vi "Create Structure ID from Structure.vi"(9 "Alphabet":string[](array[string])=["0", "1", "2", "3", "4", "5", "6", "7", "8", "9", "a", "b", "c", "d", "e", "f", "g", "h", "i", "j", "k", "l", "m", "n", "o", "p", "q", "r", "s", "t", "u", "v", "w", "x", "y", "z", "A", "B", "C", "D", "E", "F", "G", "H", "I", "J", "K", "L", "M", "N", "O", "P", "Q", "R", "S", "T", "U", "V", "W", "X", "Y", "Z"], 10 "ID Length":i32=12, 11 "Structure":T1={"Structure ID"="A3B3_strain", "Lattice vector a"=[4.67354, 0.0, 0.0], "Lattice vector b"=[0.0, 8.0948, 0.0], "Lattice vector c"=[0.0, 0.0, 23.043272], "Atoms Array"=[{"Atom Name"="Cd", "Positions (Direct)"=[[0.0, 0.3333526109234154, 0.0418710942225006], [0.5000009999999975, 0.8333529332228705, 0.0418710547186735], [0.5000009999999975, 0.166659409006074, 0.20845808075038], [0.0, 0.6666596363811387, 0.2084580241418204], [0.0, -8.44898704729e-05, 0.3751631556991639], [0.5000009999999975, 0.4999164138500652, 0.375163134357792], [0.0, 8.44898704729e-05, 0.8751631556991638], [0.5000009999999975, 0.5000855861499368, 0.8751631343577921], [0.0, 0.3333423636188632, 0.7084570241418229], [0.5000009999999975, 0.833342590993928, 0.7084570807503824], [0.5000009999999975, 0.1666490667771315, 0.5418710547186734], [0.0, 0.6666493890765864, 0.5418710942225006]], "Positions (Cartesian)"=[[0.0, 2.6984227149028626, 0.9648470131067098], [2.3367746735399884, 6.7458253238524915, 0.9648461028092771], [2.3367746735399884, 1.3490745840223677, 4.803556255328971], [0.0, 5.396476424578041, 4.803554950882535], [0.0, -0.0006839286035040309, 8.644986641154185], [2.3367746735399884, 4.0467233868335075, 8.644986149379148], [0.0, 0.0006839286035040309, 20.166622641154184], [2.3367746735399884, 4.048092802766508, 20.16662214937915], [0.0, 2.6983397650219736, 16.32516790761059], [2.3367746735399884, 6.745741605577648, 16.325169212057027], [2.3367746735399884, 1.348990865747524, 12.486482102809275], [0.0, 5.396393474697152, 12.48648301310671]]}, {"Atom Name"="Te", "Positions (Direct)"=[[0.0, 0.9999785268032801, -4.68232631346e-05], [0.5000009999999975, 0.4999797936920724, -4.67924585214e-05], [0.0, 0.3333755265141826, 0.1664730611888124], [0.5000009999999975, 0.8333756986686149, 0.1664729662126494], [0.5000009999999975, 0.1665154827798591, 0.3330835443926201], [0.0, 0.6665158170693574, 0.3330835000372194], [0.0, 0.3334861829306446, 0.833082500037222], [0.5000009999999975, 0.833486517220143, 0.8330825443926226], [0.5000009999999975, 0.16662630133138, 0.6664729662126494], [0.0, 0.6666264734858195, 0.6664730611888123], [0.0, 2.14731967198e-05, 0.4999531767368653], [0.5000009999999975, 0.5000222063079295, 0.4999532075414786]], "Positions (Cartesian)"=[[0.0, 8.094626178767191, -0.0010789611883381606], [2.3367746735399884, 4.047236433978587, -0.0010782513492573382], [0.0, 2.6986082120270054, 3.8360840296464476], [2.3367746735399884, 6.746009605582704, 3.8360818410848903], [2.3367746735399884, 1.3479095300064032, 7.67533471216322], [0.0, 5.395312236013034, 7.675333690069658], [0.0, 2.6995039535869814, 19.196946646797716], [2.3367746735399884, 6.746906659593613, 19.19694766889128], [2.3367746735399884, 1.3488065840172547, 15.357717841084892], [0.0, 5.396207977573011, 15.357720029646448], [0.0, 0.00017382123280743704, 11.52055703881166], [2.3367746735399884, 4.0475797556214275, 11.520557748650743]]}], "# of atoms"=24}) -> (3 "Structure ID":string="S9HVHL68rkOYQr")   [LabVIEW 2010]
uses:
  <vilib>/Analysis/_algsub.llb/Real Vector Norm.vi
  <vilib>/Analysis/NI_AALPro.lvlib
panel:
  out "Numeric 2":dbl=27.85452959635157
  out "Numeric":dbl=0.1091853688299409 format="%#_12g"
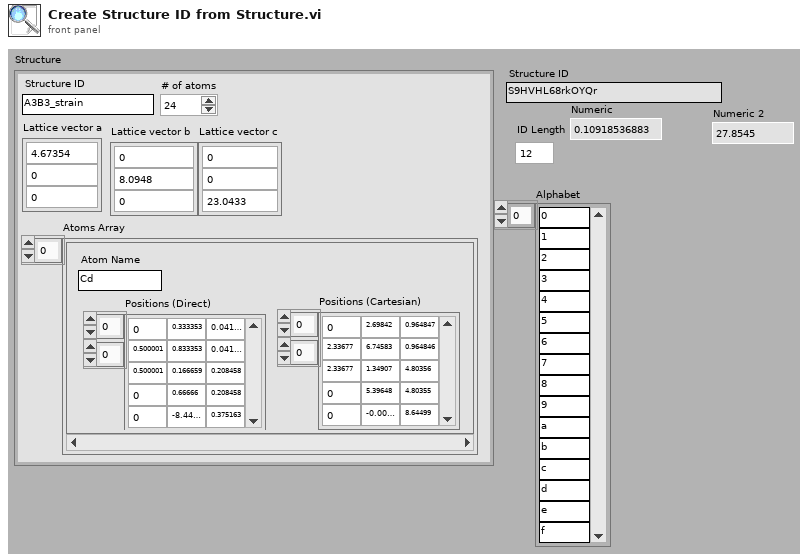
[diagram p1: front panel]
types:
  T1 = cluster{"Structure ID":string, "Lattice vector a":dbl[], "Lattice vector b":dbl[], "Lattice vector c":dbl[], "Atoms Array":cluster{"Atom Name":string, "Positions (Direct)":dbl[][], "Positions (Cartesian)":dbl[][]}[], "# of atoms":i32}
  T2 = cluster{"Atom Name":string, "Positions (Direct)":dbl[][], "Positions (Cartesian)":dbl[][]}[]
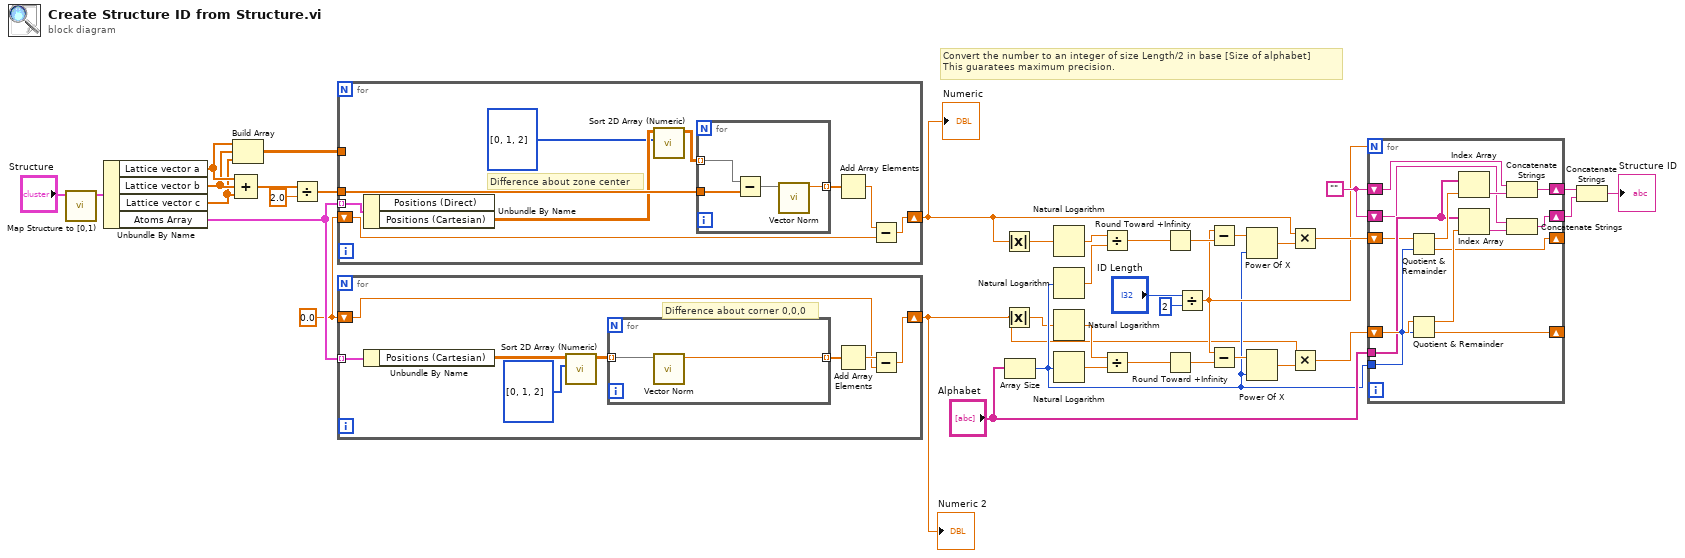
[diagram p0: block diagram]
diagram:
  w27 = ""
  w32 = 0.0
  # "Convert the number to an integer of size Length/2 in base [Size of alphabet]\nThis guaratees maximum precision."
  n1 = call "Map Structure to [0,1).vi"("Structure"="Structure") -> ("Structure mapped to [0,1)"=w1:T1)  [unwired: 10 in]
  n2 = Unbundle By Name(w1) -> ("Lattice vector a"=w6:dbl[], "Lattice vector b"=w5:dbl[], "Lattice vector c"=w4:dbl[], "Atoms Array"=w38:T2)
  n3 = Build Array(w6, w5, w4) -> (w3:dbl[][])
  n4 = Compound Arithmetic op=ADD(w6, w5, w4) -> (w36:dbl[])
  n5 = Divide(x=w36, y=2.0) -> (x/y=w35:dbl[])
  n6 = for {
    tunnel: w38 -> [w47] mode=indexing
    shift-right: [w44] -> w8
    shift-left: w32 -> [w45]
    tunnel: w35 -> [w42]
    tunnel: w3 -> [_]
    # "Difference about zone center"
    n7 = Unbundle By Name(w47) -> ("Positions (Cartesian)"=w41:dbl[][])  [unwired: 1 out]
    n8 = call "Sort 2D Array (Numeric).vi"("Sort by Cols"=i32[] [0, 1, 2], "Input Array"=w41) -> ("Output Array"=w39:dbl[][])  [unwired: 9 in]
    n9 = for {
      tunnel: [w51] -> w43 mode=indexing
      tunnel: w42 -> [w50]
      tunnel: w39 -> [w48] mode=indexing
      n10 = Subtract(x=w48, y=w50) -> (x-y=w49:dbl[])
      n11 = call-poly <vilib>:"Vector Norm.vi"("Input Vector"=w49) -> ("norm"=w51:dbl)  [unwired: 9 in, 1 out]
    }
    n12 = Add Array Elements(numeric array=w43) -> (sum=w46:dbl)
    n13 = Subtract(x=w46, y=w45) -> (x-y=w44:dbl)
  }
  "Numeric" <- w8
  n14 = for {
    tunnel: w38 -> [w59] mode=indexing
    shift-right: [w56] -> w10
    shift-left: w32 -> [w57]
    # "Difference about corner 0,0,0"
    n15 = Unbundle By Name(w59) -> ("Positions (Cartesian)"=w53:dbl[][])
    n16 = call "Sort 2D Array (Numeric).vi"("Sort by Cols"=i32[] [0, 1, 2], "Input Array"=w53) -> ("Output Array"=w52:dbl[][])  [unwired: 9 in]
    n17 = for {
      tunnel: w52 -> [w61] mode=indexing
      tunnel: [w60] -> w55 mode=indexing
      n18 = call-poly <vilib>:"Vector Norm.vi"("Input Vector"=w61) -> ("norm"=w60:dbl)  [unwired: 9 in, 1 out]
    }
    n19 = Add Array Elements(numeric array=w55) -> (sum=w58:dbl)
    n20 = Subtract(x=w58, y=w57) -> (x-y=w56:dbl)
  }
  "Numeric 2" <- w10
  n21 = Absolute Value(x=w8) -> (abs(x)=w7:dbl)
  n22 = Absolute Value(x=w10) -> (abs(x)=w9:dbl)
  n23 = Array Size(array="Alphabet") -> (size(s)=w11:i32)
  n24 = Natural Logarithm(1:w7) -> (0:w23:dbl)
  n25 = Natural Logarithm(1:w11) -> (0:w24:dbl)
  n26 = Natural Logarithm(1:w9) -> (0:w17:dbl)
  n27 = Natural Logarithm(1:w11) -> (0:w16:dbl)
  n28 = Divide(x=w23, y=w24) -> (x/y=w22:dbl)
  n29 = Divide(x=w17, y=w16) -> (x/y=w18:dbl)
  n30 = Round Toward +Infinity(x=w22) -> (ceil(x): smallest int >= x=w25:dbl)
  n31 = Round Toward +Infinity(x=w18) -> (ceil(x): smallest int >= x=w15:dbl)
  n32 = Divide(x="ID Length", y=2) -> (x/y=w13:dbl)
  n33 = Subtract(x=w13, y=w25) -> (x-y=w20:dbl)
  n34 = Subtract(x=w13, y=w15) -> (x-y=w19:dbl)
  n35 = Power Of X(1:w11, 2:w20) -> (0:w26:dbl)
  n36 = Power Of X(1:w11, 2:w19) -> (0:w14:dbl)
  n37 = Multiply(x=w8, y=w26) -> (x*y=w21:dbl)
  n38 = Multiply(x=w10, y=w14) -> (x*y=w12:dbl)
  n39 = for {
    N: w13 -> [_]
    tunnel: w11 -> [w64]
    tunnel: "Alphabet" -> [w70]
    shift-right: [w63] -> _
    shift-left: w21 -> [w62]
    shift-right: [w73] -> w30
    shift-left: w27 -> [w72]
    shift-right: [w68] -> _
    shift-left: w12 -> [w71]
    shift-right: [w66] -> w29
    shift-left: w27 -> [w65]
    n40 = Quotient & Remainder(x=w62, y=w64) -> (x-y*floor(x/y)=w75:dbl, floor(x/y)=w63:dbl)
    n41 = Quotient & Remainder(x=w71, y=w64) -> (x-y*floor(x/y)=w69:dbl, floor(x/y)=w68:dbl)
    n42 = Index Array(array=w70, index=w75) -> (element=w74:string)
    n43 = Index Array(array=w70, index=w69) -> (element=w67:string)
    n44 = Concatenate Strings(w72, w74) -> (w73:string)
    n45 = Concatenate Strings(w65, w67) -> (w66:string)
  }
  n46 = Concatenate Strings(w30, w29) -> (→"Structure ID":string)
